vi "Output.vi"(9 "Module Info In":T1, 11 "Engine Tags In":T3) -> (1 "Module Info Out":T1, 3 "Engine Tags Out":T3)   [LabVIEW 2013]
doc: "This VI calls the output method of any modules specified using the 'Output Method Indices' if the 'Execute?' flag for the method is TRUE. It also exchanges the data necessary for that method with the data in the main engine tags. Any errors that occur are stored to be handled at the end of the engine's execution."
uses:
  <vilib>/NI/Tag Bus/table/data table.ctl
  Module Execution Info.ctl
  <vilib>/NI/Tag Bus Module Framework/runtime/TBM module execution interface.lvclass
  Data Table with Transfer Spec.ctl
  <vilib>/NI/Tag Bus/table/transfer specification.ctl
  <vilib>/NI/Tag Bus/tag/Data Type.ctl
  Configuration/Module Decimation.ctl
  Configuration/Module Error Configuration.ctl
  Configuration/Error Actions By Category.ctl
  <vilib>/NI/Tag Bus Module Framework/runtime/error classification.ctl
  Configuration/Error Actions.ctl
  error responses.ctl
  Configuration/error options.ctl
  <vilib>/NI/Tag Bus/table/data table.lvlib
  <vilib>/NI/Tag Bus/tag/tag descriptor.lvclass
  Configuration/Standard Engine Configuration.lvclass
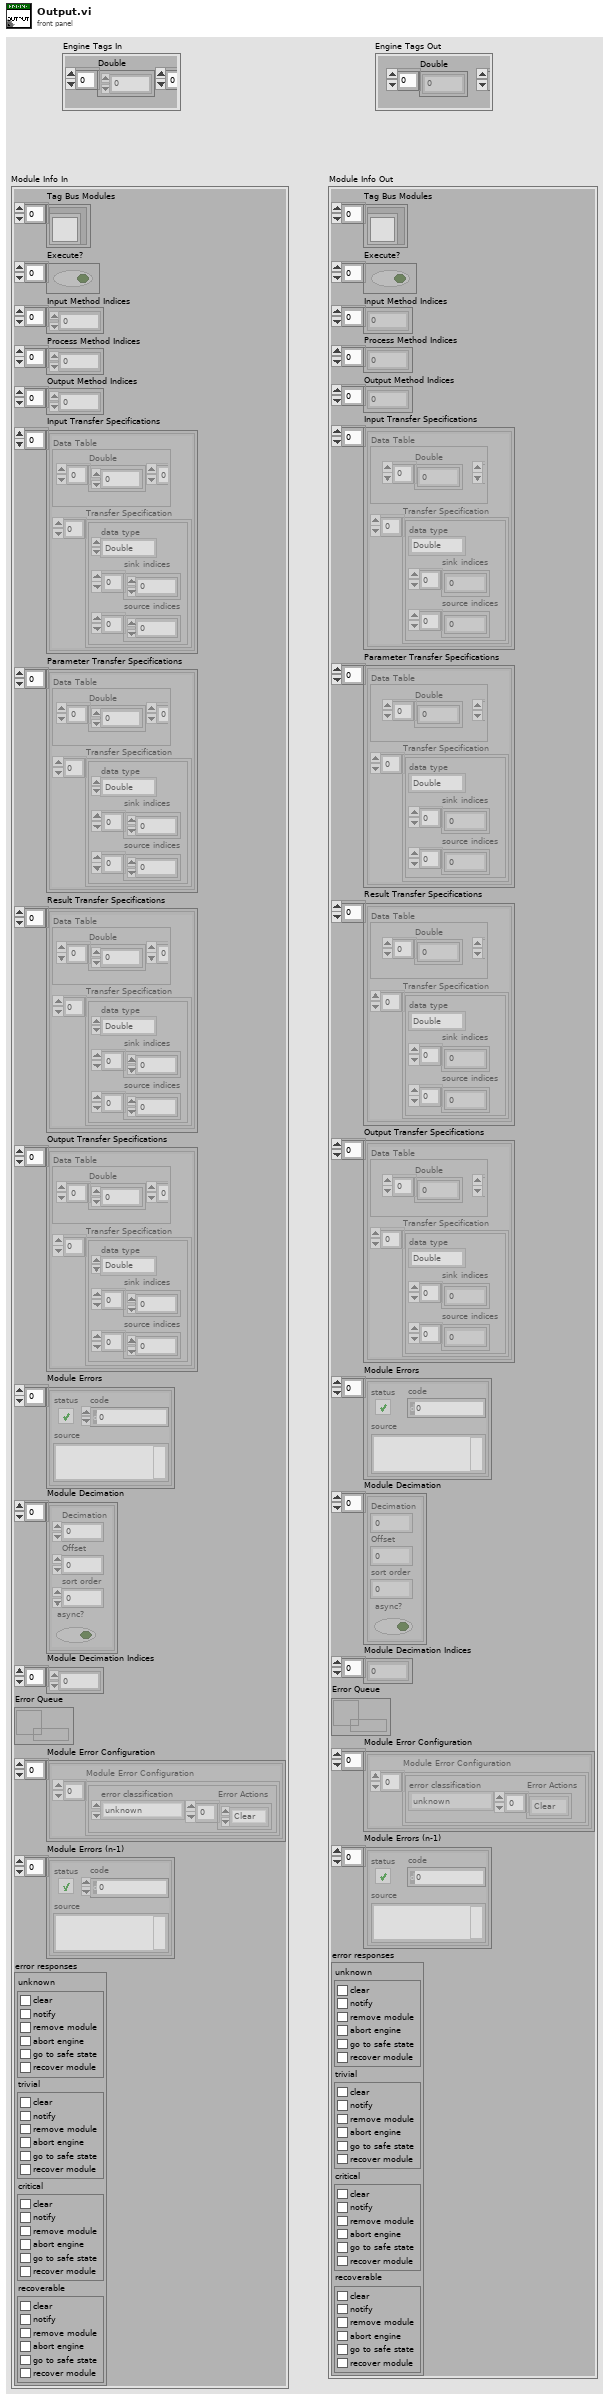
[diagram p1: front panel]
types:
  T1 = typedef "Module Execution Info.ctl" = cluster{"Tag Bus Modules":refnum<class "TBM module execution interface.lvclass">[], "Execute?":bool[], "Input Method Indices":i32[], "Process Method Indices":i32[], "Output Method Indices":i32[], "Input Transfer Specifications":T2[], "Parameter Transfer Specifications":T2[], "Result Transfer Specifications":T2[], "Output Transfer Specifications":T2[], "Module Errors":errorcluster[], "Module Decimation":T6[], "Module Decimation Indices":i32[], "Error Queue":refnum<queue>, "Module Error Configuration":T7[], "Module Errors (n-1)":errorcluster[], "error responses":T11}
  T2 = typedef "Data Table with Transfer Spec.ctl" = cluster{"Data Table":T3, "Transfer Specification":T4[]}
  T3 = typedef "tag bus.lvlib/data table.lvlib/data table.ctl" = cluster{"Double":dbl[], "Single":sgl[], "I64":i64[], "I32":i32[], "I16":i16[], "I8":i8[], "U64":u64[], "U32":u32[], "U16":u16[], "U8":u8[], "Boolean":bool[], "String":string[], "Array of Double":cluster{"DBL Array":dbl[]}[], "Array of Single":cluster{"SGL Array":sgl[]}[], "Array of I64":cluster{"I64 Array":i64[]}[], "Array of I32":cluster{"I32 Array":i32[]}[], "Array of I16":cluster{"I16 Array":i16[]}[], "Array of I8":cluster{"I8 Array":i8[]}[], "Array of U64":cluster{"U64 Array":u64[]}[], "Array of U32":cluster{"U32 Array":u32[]}[], "Array of U16":cluster{"U16 Array":u16[]}[], "Array of U8":cluster{"U8 Array":u8[]}[], "Array of Boolean":cluster{"Boolean Array":bool[]}[], "Array of String":cluster{"String Array":string[]}[]}
  T4 = typedef "tag bus.lvlib/data table.lvlib/transfer specification.ctl" = cluster{"data type":T5, "sink indices":i32[], "source indices":i32[]}
  T5 = typedef "tag bus.lvlib/tag descriptor.lvclass/Data Type.ctl" = enum16{"Double", "Single", "I64", "I32", "I16", "I8", "U64", "U32", "U16", "U8", "Boolean", "String", "Array of Double", "Array of Single", "Array of I64", "Array of I32", "Array of I16", "Array of I8", "Array of U64", "Array of U32", "Array of U16", "Array of U8", "Array of Boolean", "Array of String"}
  T6 = typedef "Standard Engine Configuration.lvclass/Module Decimation.ctl" = cluster{"Decimation":u16, "Offset":u16, "sort order":i32, "async?":bool}
  T7 = typedef "Standard Engine Configuration.lvclass/Module Error Configuration.ctl" = cluster{"Module Error Configuration":T8[]}
  T8 = typedef "Standard Engine Configuration.lvclass/Error Actions By Category.ctl" = cluster{"error classification":T9, "Error Actions":T10[]}
  T9 = typedef "TBM module execution interface.lvclass/error classification.ctl" = enum16{"unknown", "none", "trivial", "recoverable", "critical"}
  T10 = typedef "Standard Engine Configuration.lvclass/Error Actions.ctl" = enum16{"Clear", "Notify", "Stop Component", "Stop Engine", "Safe State", "Attempt Recovery"}
  T11 = typedef "Standard Engine Configuration.lvclass/error responses.ctl" = cluster{"unknown":T12, "trivial":T12, "critical":T12, "recoverable":T12}
  T12 = typedef "Standard Engine Configuration.lvclass/error options.ctl" = cluster{"clear":bool, "notify":bool, "remove module":bool, "abort engine":bool, "go to safe state":bool, "recover module":bool}
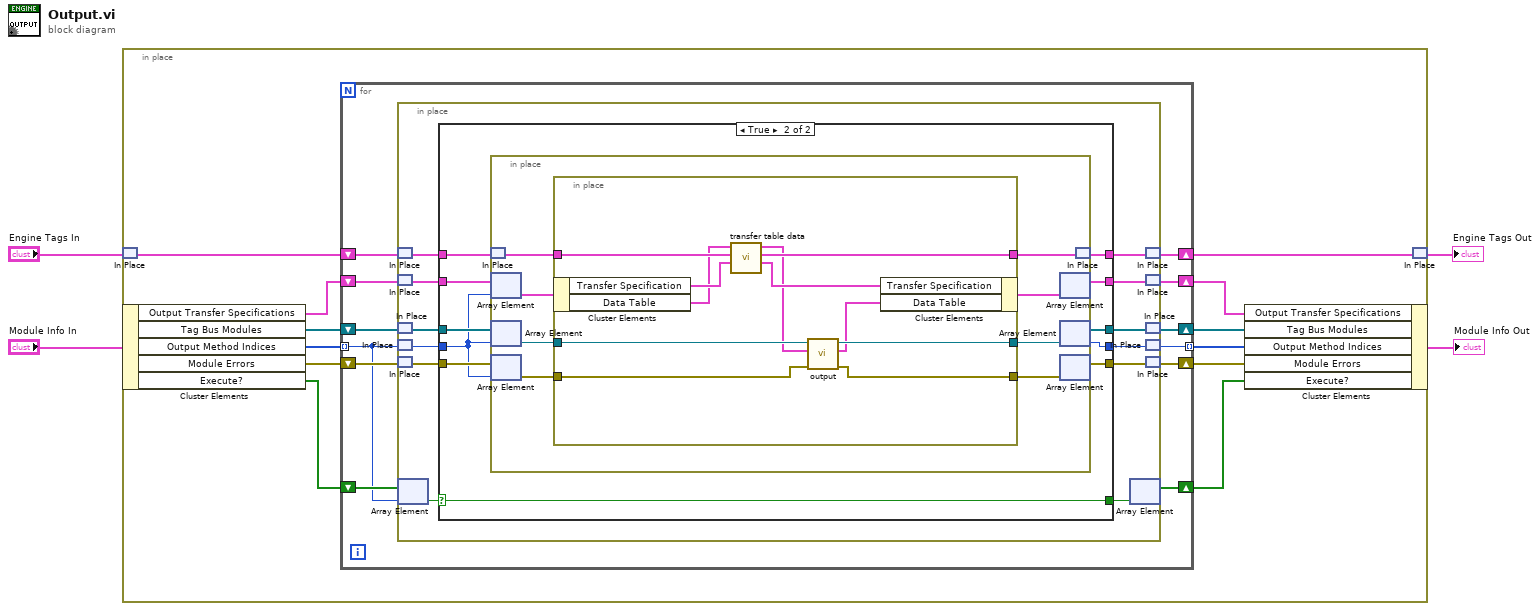
[diagram p0: block diagram]
diagram:
  n1 = in-place {
    n2 = in-place-match #1("Engine Tags In") -> (w15:T3)
    n3 = in-place-cluster #2("Module Info In") -> ("Output Transfer Specifications"=w13:T2[], "Tag Bus Modules"=w10:refnum<class "TBM module execution interface.lvclass">[], "Output Method Indices"=w16:i32[], "Module Errors"=w12:errorcluster[], "Execute?"=w6:bool[])
    n4 = for {
      shift-right: [w21] -> w9
      shift-left: w10 -> [w22]
      tunnel: w16 -> [w18] mode=indexing
      shift-right: [w25] -> w14
      shift-left: w15 -> [w26]
      shift-right: [w23] -> w11
      shift-left: w13 -> [w24]
      shift-right: [w19] -> w8
      shift-left: w12 -> [w20]
      tunnel: [w17] -> w7 mode=indexing
      shift-right: [w27] -> w5
      shift-left: w6 -> [w28]
      n5 = in-place {
        n6 = in-place-match #3(w26) -> (w38:T3)
        n7 = in-place-match #4(w24) -> (w36:T2[])
        n8 = in-place-match #5(w22) -> (w34:refnum<class "TBM module execution interface.lvclass">[])
        n9 = in-place-match #6(w18) -> (w30:i32)
        n10 = in-place-match #7(w20) -> (w32:errorcluster[])
        n11 = in-place-array #8(w28, w18) -> (w40:bool)
        n12 = case shown="True" w40 {
          selector: w40 -> [w41 w47]
          tunnel: w38 -> [w46 w57]
          tunnel: [w46 w56] -> w37
          tunnel: w36 -> [w45 w55]
          tunnel: w34 -> [w44 w54]
          tunnel: w32 -> [w42 w53]
          tunnel: [w45 w52] -> w35
          tunnel: [w42 w51] -> w31
          tunnel: [w44 w50] -> w33
          tunnel: w30 -> [w43 w49]
          tunnel: [w43 w48] -> w29
          tunnel: [w41 w47] -> w39
          frame False {
          }
          frame True {
            n13 = in-place {
              n14 = in-place-match #9(w57) -> (w61:T3)
              n15 = in-place-array #10(w55, w49) -> (w59:T2)
              n16 = in-place-array #11(w54, w49) -> (w65:refnum<class "TBM module execution interface.lvclass">)
              n17 = in-place-array #12(w53, w49) -> (w63:errorcluster)
              n18 = in-place {
                in-place-border: w65 -> [w76]
                in-place-border: [w75] -> w64
                in-place-border: w63 -> [w74]
                in-place-border: [w73] -> w62
                in-place-border: w61 -> [w72]
                in-place-border: [w71] -> w60
                n19 = in-place-cluster #13(w59) -> ("Transfer Specification"=w70:T4[], "Data Table"=w68:T3)
                n20 = call <vilib>:"transfer table data.vi"("transfer specification in"=w70, "data table source in"=w72, "data table sink in"=w68) -> ("transfer specification out"=w69:T4[], "data table source out"=w71:T3, "data table sink out"=w67:T3)  [unwired: 6 in]
                n21 = call-dynamic "output.vi"("error in"=w74, "output data"=w67, "module in"=w76) -> ("error out"=w73:errorcluster, "output allocation"=w66:T3, "module out"=w75:refnum<class "TBM module execution interface.lvclass">)  [unwired: 6 in]
                n22 = in-place-cluster #13("Transfer Specification"=w69, "Data Table"=w66) -> (w58:T2)
              }
              n23 = in-place-array #10(w58) -> (w52:T2[])  [unwired: 1 out]
              n24 = in-place-array #11(w64) -> (w50:refnum<class "TBM module execution interface.lvclass">[], w48:i32)
              n25 = in-place-array #12(w62) -> (w51:errorcluster[])  [unwired: 1 out]
              n26 = in-place-match #9(w60) -> (w56:T3)
            }
          }
        }
        n27 = in-place-array #8(w39) -> (w27:bool[])  [unwired: 1 out]
        n28 = in-place-match #3(w37) -> (w25:T3)
        n29 = in-place-match #4(w35) -> (w23:T2[])
        n30 = in-place-match #5(w33) -> (w21:refnum<class "TBM module execution interface.lvclass">[])
        n31 = in-place-match #6(w29) -> (w17:i32)
        n32 = in-place-match #7(w31) -> (w19:errorcluster[])
      }
    }
    n33 = in-place-cluster #2("Output Transfer Specifications"=w11, "Tag Bus Modules"=w9, "Output Method Indices"=w7, "Module Errors"=w8, "Execute?"=w5) -> (→"Module Info Out":T1)
    n34 = in-place-match #1(w14) -> (→"Engine Tags Out":T3)
  }
